vi "TDMS_NotesViewer.vi"() -> ()   [LabVIEW 2019]
panel:
  out "Experiment Notes":string
  in  "Files":i32(listbox)
  in  "Experiment Path":path
  in  "OK":bool
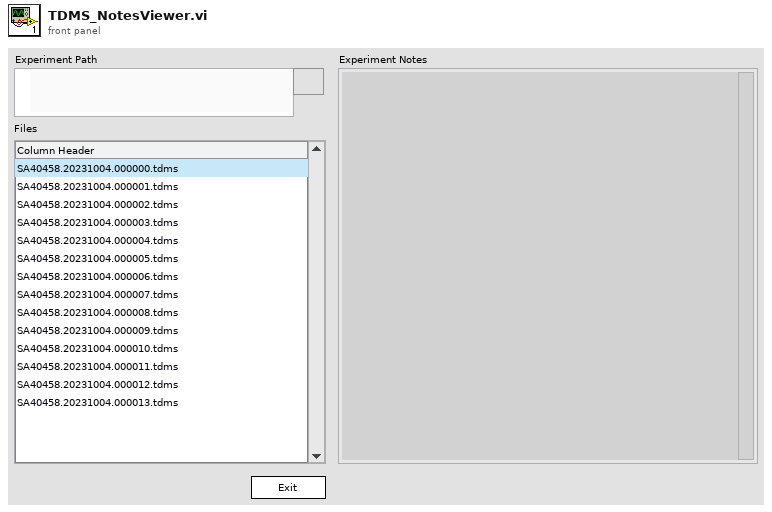
[diagram p1: front panel]
types:
  T1 = enum32{"Invalid", "Standard", "Closed", "Hidden", "Minimized", "Maximized"}
  T2 = enum32{"invalid app kind", "Development System", "Run Time System", "Student Edition", "Embedded LabVIEW", "Evaluation", "Custom"}
  T3 = cluster{"Core":cluster{"Current VI Reference":refnum<vi>, "Close Panel on Exit?":bool}, "Your Boolean data":bool, "Your string data":string, "File list":string[], "Experiment Path":path}
  T4 = cluster{"Current VI Reference":refnum<vi>, "Close Panel on Exit?":bool}
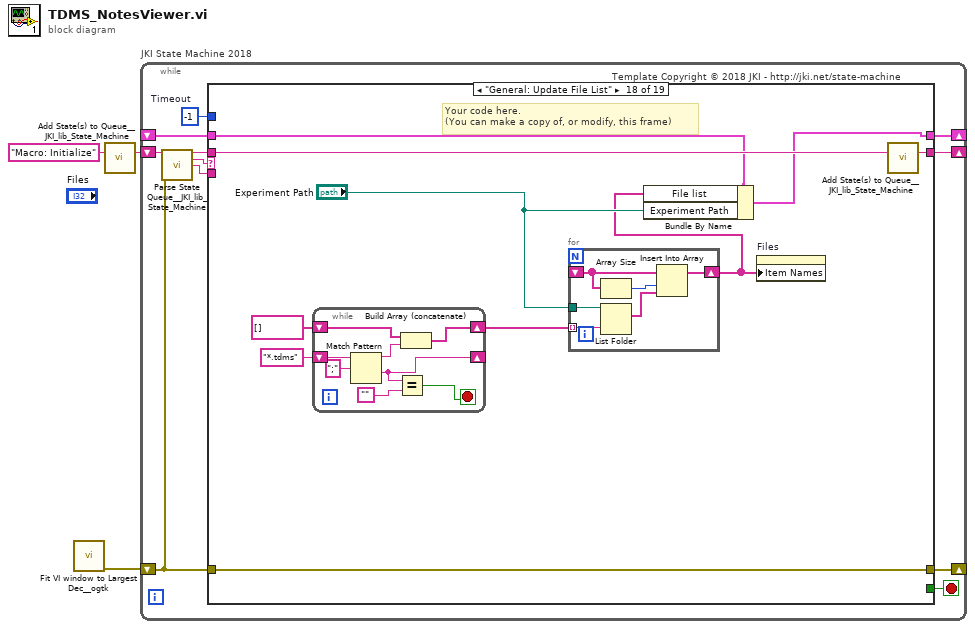
[diagram p0: block diagram]
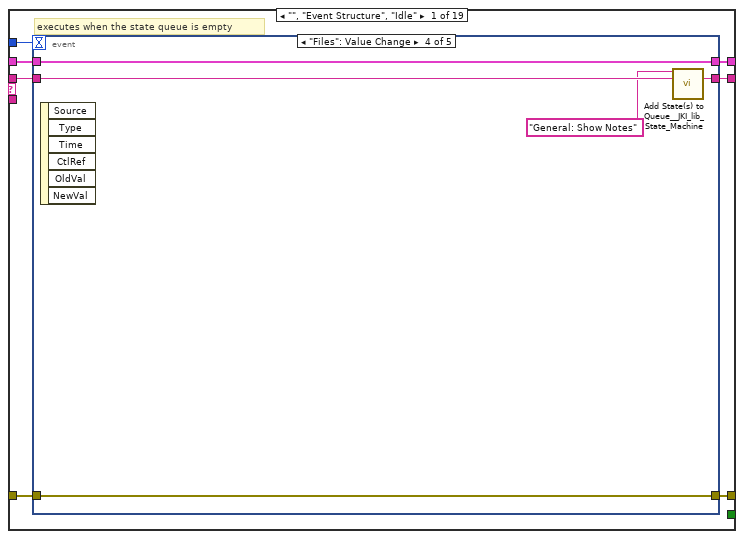
[diagram p2: hidden frame]
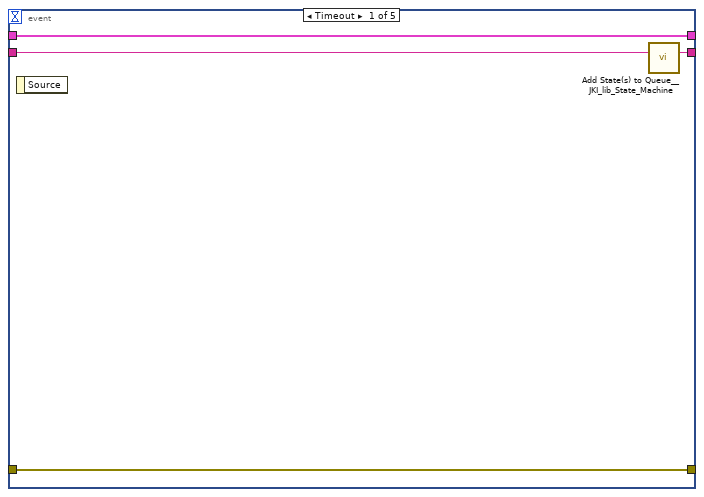
[diagram p3: hidden frame]
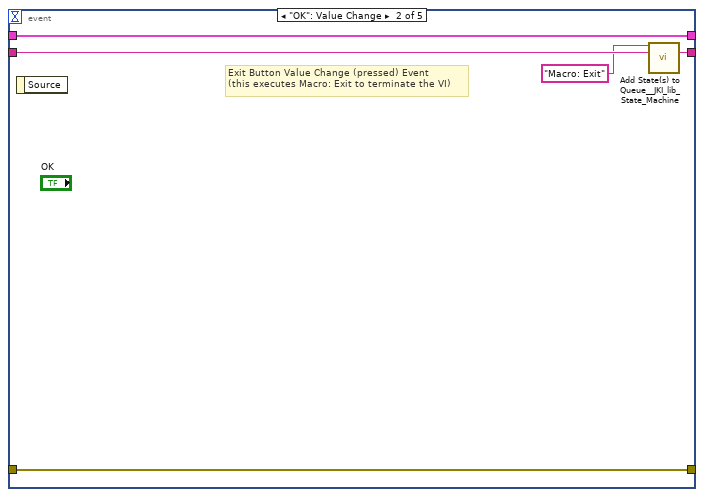
[diagram p4: hidden frame]
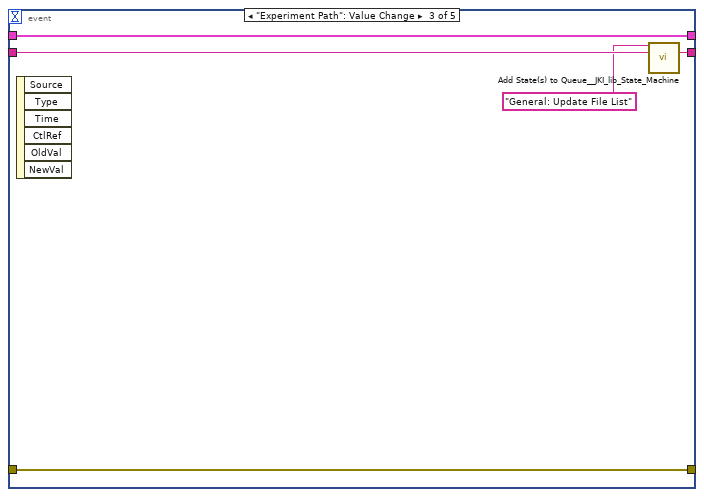
[diagram p5: hidden frame]
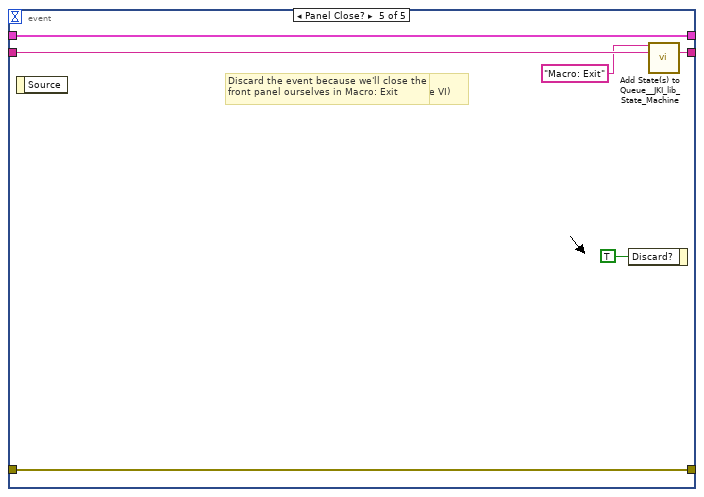
[diagram p6: hidden frame]
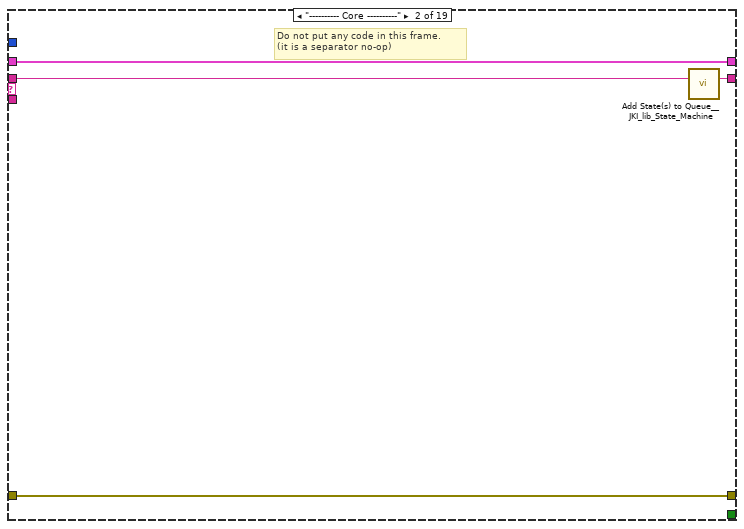
[diagram p7: hidden frame]
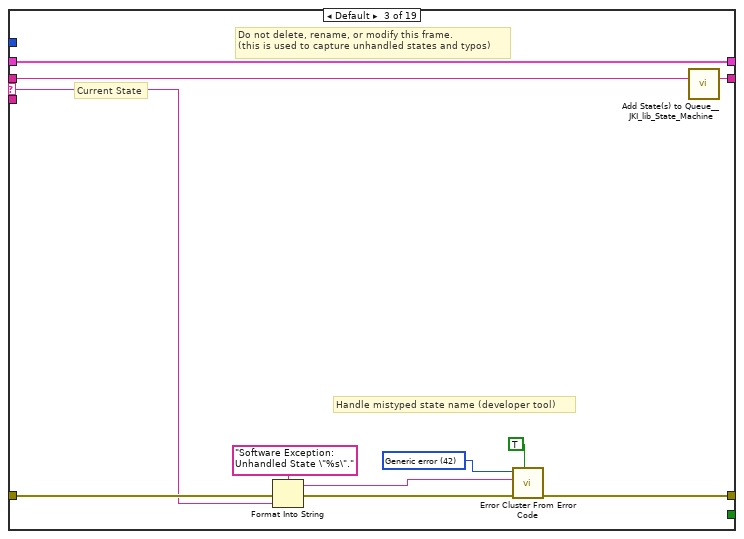
[diagram p8: hidden frame]
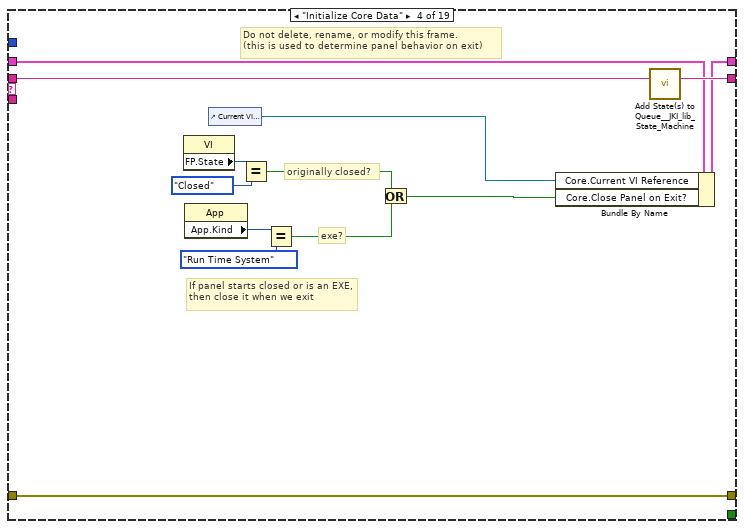
[diagram p9: hidden frame]
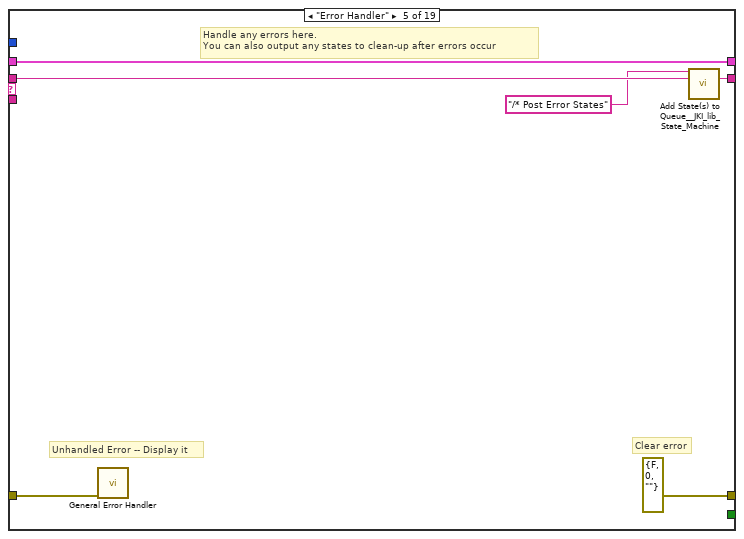
[diagram p10: hidden frame]
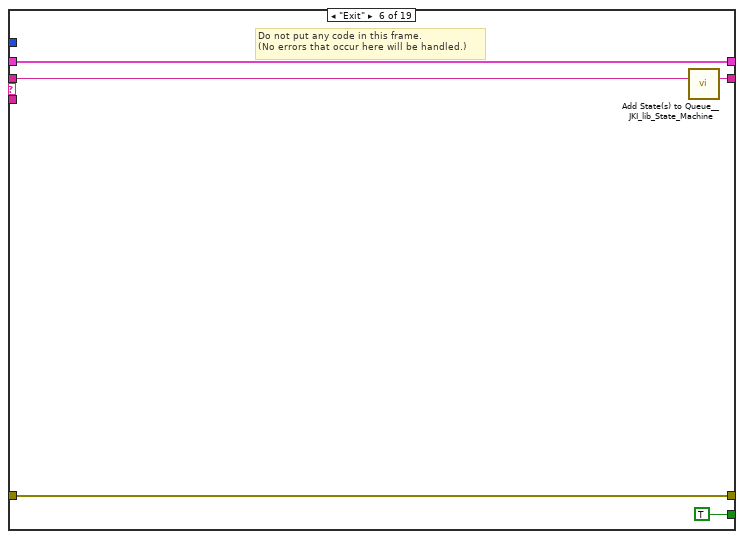
[diagram p11: hidden frame]
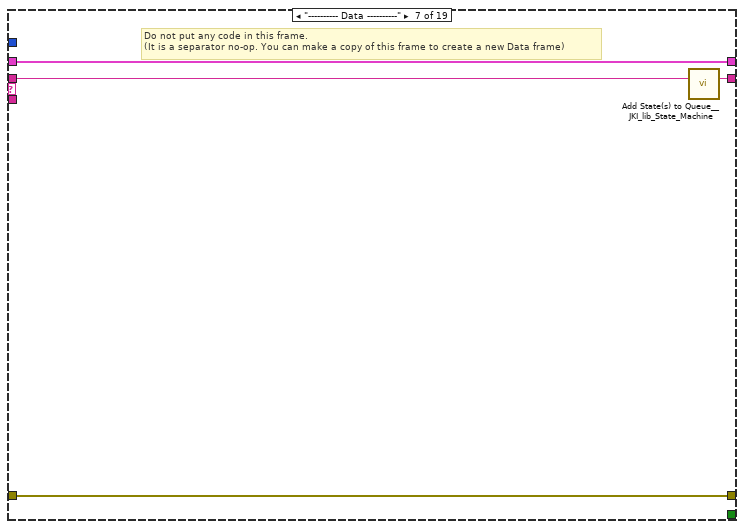
[diagram p12: hidden frame]
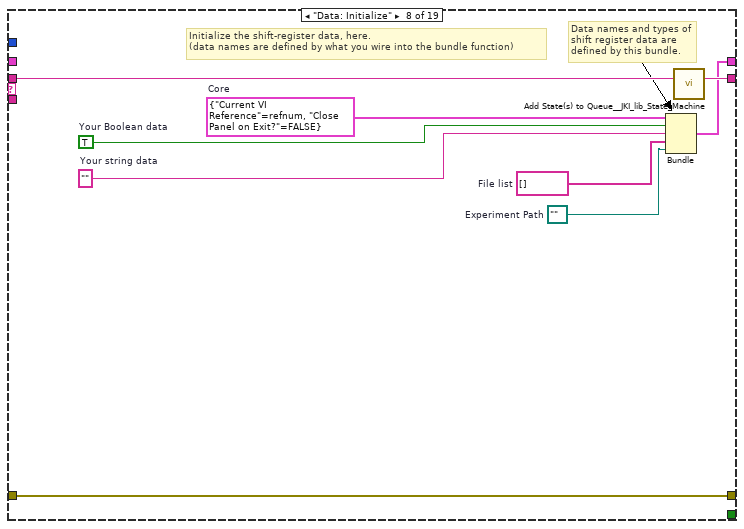
[diagram p13: hidden frame]
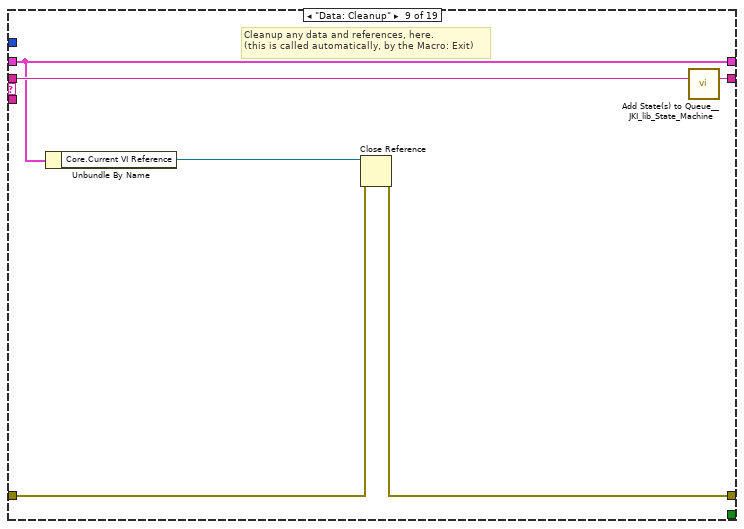
[diagram p14: hidden frame]
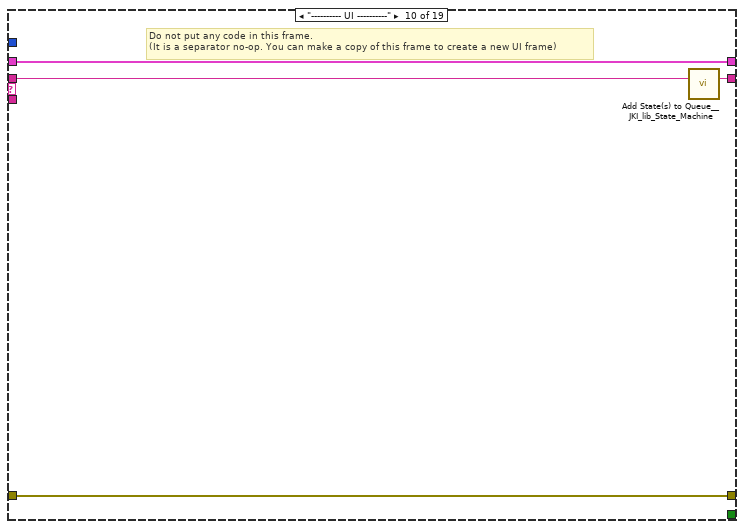
[diagram p15: hidden frame]
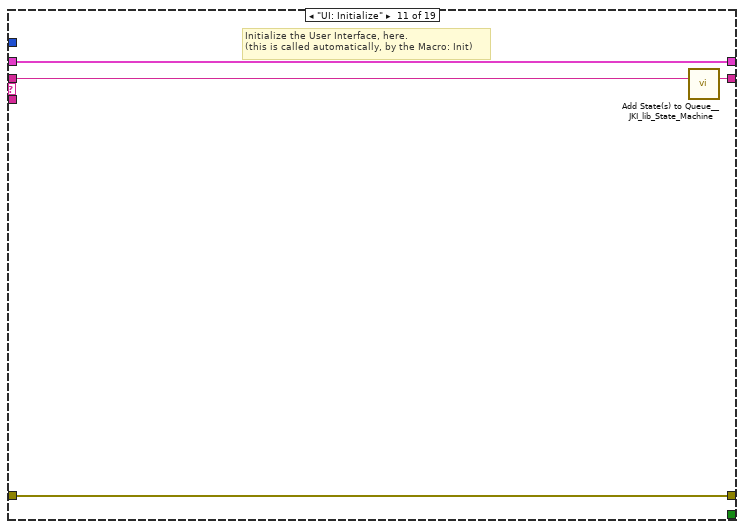
[diagram p16: hidden frame]
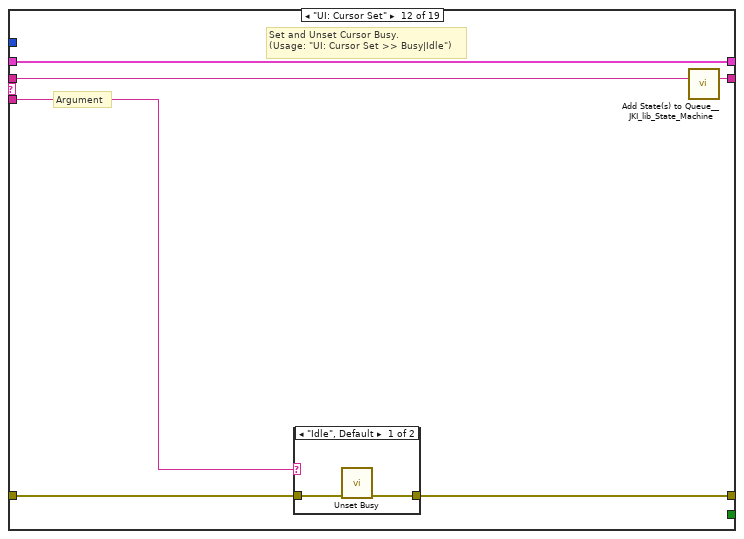
[diagram p17: hidden frame]
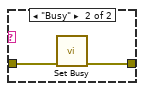
[diagram p18: hidden frame]
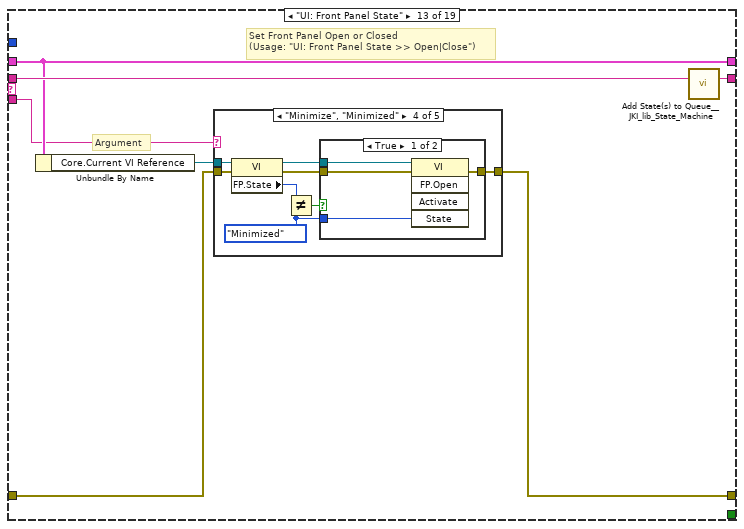
[diagram p19: hidden frame]
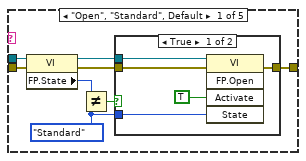
[diagram p20: hidden frame]
diagram:
  n1 = call <userlib>:"Fit VI window to Largest Dec__ogtk.vi"() -> ("error out"=w1:errorcluster)  [unwired: 6 in, 1 out]
  n2 = call <vilib>:"Add State(s) to Queue__JKI_lib_State_Machine.vi"("State(s) in (\"\")"="Macro: Initialize") -> ("States Out"=w3:string)  [unwired: 14 in]
  n3 = while "JKI State Machine 2018" {
    shift-right: [w7] -> _
    shift-left: _ -> [w6]
    shift-right: [w10] -> _
    shift-left: w1 -> [w4]
    shift-right: [w9] -> _
    shift-left: w3 -> [w11]
    stop <- w8 stop-if-true
    w5 = -1  # Timeout
    # "Template Copyright © 2018 JKI - http://jki.net/state-machine"
    n4 = call <vilib>:"Parse State Queue__JKI_lib_State_Machine.vi"("State Queue"=w11, "Error In (no error)"=w4) -> ("Remaining States"=w13:string, "Current State"=w14:string, "Arguments"=w12:string)  [unwired: 11 in]
    n5 = case shown="\"General: Update File List\"" w14 {
      selector: w14 -> [_ _ w51 _ _ _ _ _ _ _ _ _ _ _ _ _ _ _ _]
      tunnel: w13 -> [w21 w50 w55 w74 w80 w85 w89 w98 w104 w108 w112 w118 w129 w198 w203 w213 w217 w227 w259]
      tunnel: w12 -> [_ _ _ _ _ _ _ _ _ _ _ w113 w123 _ _ _ _ _ _]
      tunnel: w6 -> [w19 w47 w53 w67 w77 w83 w86 _ w99 w105 w110 w116 w125 w195 w200 w210 w214 w225 w256]
      tunnel: [w18 w48 w57 w71 errorcluster {"status"=FALSE, "code"=0, "source"=""} ("error out") w82 w87 w95 w100 w106 w109 w114 w126 w196 w201 w211 w215 w218 w257] -> w10
      tunnel: w4 -> [w17 w48 w56 w71 w76 w82 w87 w95 w101 w106 w109 w115 w127 w196 w201 w211 w215 w218 w257]
      tunnel: [w20 w49 w54 w73 w79 w84 w88 w97 w103 w107 w111 w117 w128 w197 w202 w212 w216 w226 w258] -> w9
      tunnel: [_ _ _ _ _ TRUE _ _ _ _ _ _ _ _ _ _ _ _ _] -> w8
      tunnel: [w16 w47 w53 w72 w77 w83 w86 w96 w99 w105 w110 w116 w125 w195 w200 w210 w214 w224 w256] -> w7
      tunnel: w5 -> [w15 _ _ _ _ _ _ _ _ _ _ _ _ _ _ _ _ _ _]
      frame "", "Event Structure", "Idle" {
        # "executes when the state queue is empty"
        n6 = event shown="[3] \"Files\": Value Change" {
          selector: _ -> [_ _ _ _ _]
          dyn-events: _ -> [_ _ _ _ _]
          timeout: w15 -> [_ _ _ _ _]
          tunnel: w21 -> [w25 w30 w35 w40 w46]
          tunnel: [w24 w29 w34 w39 w45] -> w20
          tunnel: w19 -> [w22 w27 w32 w37 w43]
          tunnel: [w23 w28 w33 w38 w44] -> w18
          tunnel: w17 -> [w23 w28 w33 w38 w44]
          tunnel: [w22 w27 w32 w37 w43] -> w16
          event Timeout {
            n7 = event-data() -> ()  [unwired: 1 in, 1 out]
            n8 = call <vilib>:"Add State(s) to Queue__JKI_lib_State_Machine.vi"("State(s) in (\"\")"=w25) -> ("States Out"=w24:string)  [unwired: 14 in]
          }
          event "OK": Value Change {
            # "Exit Button Value Change (pressed) Event\n(this executes Macro: Exit to terminate the VI)"
            n9 = event-data() -> ()  [unwired: 1 in, 1 out]
            n10 = call <vilib>:"Add State(s) to Queue__JKI_lib_State_Machine.vi"("State(s) in Front (\"\")"="Macro: Exit", "State(s) in (\"\")"=w30) -> ("States Out"=w29:string)  [unwired: 13 in]
          }
          event "Experiment Path": Value Change {
            n11 = event-data() -> ()  [unwired: 1 in, 6 out]
            n12 = call <vilib>:"Add State(s) to Queue__JKI_lib_State_Machine.vi"("State(s) in Front (\"\")"="General: Update File List", "State(s) in (\"\")"=w35) -> ("States Out"=w34:string)  [unwired: 13 in]
          }
          event "Files": Value Change {
            n13 = event-data() -> ()  [unwired: 1 in, 6 out]
            n14 = call <vilib>:"Add State(s) to Queue__JKI_lib_State_Machine.vi"("State(s) in Front (\"\")"="General: Show Notes", "State(s) in (\"\")"=w40) -> ("States Out"=w39:string)  [unwired: 13 in]
          }
          event Panel Close? {
            # "Discard the event because we'll close the front panel ourselves in Macro: Exit"
            # "Close Panel button (pressed) Event\n(this executes Macro: Exit to terminate the VI)"
            n15 = event-data() -> ()  [unwired: 1 in, 1 out]
            n16 = event-data("Discard?"=TRUE) -> ()  [unwired: 1 in, 1 out]
            n17 = call <vilib>:"Add State(s) to Queue__JKI_lib_State_Machine.vi"("State(s) in Front (\"\")"="Macro: Exit", "State(s) in (\"\")"=w46) -> ("States Out"=w45:string)  [unwired: 13 in]
          }
        }
      }
      frame "---------- Core ----------" {
        # "Do not put any code in this frame.\n(it is a separator no-op)"
        n18 = call <vilib>:"Add State(s) to Queue__JKI_lib_State_Machine.vi"("State(s) in (\"\")"=w50) -> ("States Out"=w49:string)  [unwired: 14 in]
      }
      frame Default {
        w60 = 42 items=["No error", "Argument error", "Memory is full", "Out of zone", "End of file", "File already open", "Generic file I/O error", "File not found", "File permission error", "Disk is full", "Duplicate path", "Too many files open", "System feature not enabled", "Resource file not found", "Cannot add resource", "Resource not found", "Image not found", "Image memory error", "Pen does not exist", "Config type invalid", "Config token not found", "Config parse error", "Config memory error", "Bad external code format", "Bad external code offset", "External code not present", "Null window", "Destroy window error", "Null menu", "Print aborted", "Bad print record", "Print driver error", "Windows error during printing", "Memory error during printing", "Print dialog error", "Generic print error", "Invalid device refnum", "Device not found", "Device parameter error", "Device unit error", "Cannot open device", "Device call aborted", "Generic error", "Cancelled by user", "Object ID too low", "Object ID too high", "Object not in heap", "Unknown heap", "Unknown object (invalid DefProc)", "Unknown object (DefProc not in table)", "Message out of range", "Invalid (null) method", "Unknown message", "Manager call not supported", "Bad address", "Network operation in progress", "Network operation timed out", "Connection is busy", "Network attribute not supported", "Network error", "Address in use", "System out of memory", "Connection aborted", "Connection refused", "Not connected", "Already connected", "Connection closed", "Initialization error (interapplication manager)", "Bad occurrence", "Wait on unbound occurrence handler", "Occurrence queue overflow", "Datalog type conflict", "Unused", "Unrecognized type (interapplication manager)", "Memory corrupt", "Failed to make temporary DLL", "Old CIN version", "Drag socket not found", "Failed to load drop-object", "Failed to register OLE object", "Failed to release OLE object", "Format specifier type mismatch", "Unknown format specifier", "Too few format specifiers", "Too many format specifiers", "Scan failed", "Newer CIN version", "Error converting to variant", "Runtime menu error", "Password tampered", "Variant attribute not found", "Incompatible variant data type", "Event data is not available", "Event Store is not present", "Occurrence is not found", "Event Queue is not created", "Event info is not available", "Refnum passed is NULL", "Error retrieving Class GUID", "Error retrieving CoClass GUID", "Error retrieving TypeLib GUID.", "Bad built application magic bytes.", "Specific driver is different from the specific driver associated with the Logical Name.", "There is no session opened to the class driver.", "Max Error", "MAX - Error with config objects", "MAX - Error loading configuration", "MAX - Group not supported"]
        # "Current State"
        # "Do not delete, rename, or modify this frame.\n(this is used to capture unhandled states and typos)"
        # "Handle mistyped state name (developer tool)"
        n19 = Format Into String(format string="Software Exception: Unhandled State \"%s\"." ("message"), error in=w56, w51) -> (resulting string=w59:string, error out=w58:errorcluster)  [unwired: 1 in]
        n20 = call <vilib>:"Error Cluster From Error Code.vi"("show call chain? (False)"=TRUE, "error in (no error)"=w58, "error message (\"\")"=w59, "error code (0)"=w60) -> ("error out"=w57:errorcluster)  [unwired: 5 in]
        n21 = call <vilib>:"Add State(s) to Queue__JKI_lib_State_Machine.vi"("State(s) in (\"\")"=w55) -> ("States Out"=w54:string)  [unwired: 14 in]
      }
      frame "Initialize Core Data" {
        # "Do not delete, rename, or modify this frame.\n(this is used to determine panel behavior on exit)"
        # "originally closed?"
        # "exe?"
        # "If panel starts closed or is an EXE, then close it when we exit"
        n22 = property class="VI"() -> ("FP.State"=w64:T1)  [unwired: 2 in, 2 out]
        n23 = property class="App"() -> ("App.Kind"=w70:T2)  [unwired: 2 in, 2 out]
        n24 = control-ref of="Current VI Reference"() -> (w65:refnum<vi>)
        n25 = Equal?(x=w64, y=T1."Closed" ("Front Panel Window:State")) -> (x = y?=w62:bool)
        n26 = Equal?(x=w70, y=T2."Run Time System" ("Application:Kind")) -> (x = y?=w68:bool)
        n27 = Or(x=w62, y=w68) -> (x .or. y?=w66:bool)
        n28 = Bundle By Name(cluster=w67, "Core.Current VI Reference"=w65, "Core.Close Panel on Exit?"=w66) -> (w72:T3)
        n29 = call <vilib>:"Add State(s) to Queue__JKI_lib_State_Machine.vi"("State(s) in (\"\")"=w74) -> ("States Out"=w73:string)  [unwired: 14 in]
      }
      frame "Error Handler" {
        # "Unhandled Error -- Display it"
        # "Handle any errors here.\nYou can also output any states to clean-up after errors occur"
        # "Clear error"
        n30 = call <vilib>:"General Error Handler.vi"("error in (no error)"=w76) -> ()  [unwired: 10 in, 5 out]
        n31 = call <vilib>:"Add State(s) to Queue__JKI_lib_State_Machine.vi"("State(s) in Front (\"\")"="/* Post Error States", "State(s) in (\"\")"=w80) -> ("States Out"=w79:string)  [unwired: 13 in]
      }
      frame "Exit" {
        # "Do not put any code in this frame.\n(No errors that occur here will be handled.)"
        n32 = call <vilib>:"Add State(s) to Queue__JKI_lib_State_Machine.vi"("State(s) in (\"\")"=w85) -> ("States Out"=w84:string)  [unwired: 14 in]
      }
      frame "---------- Data ----------" {
        # "Do not put any code in this frame.\n(It is a separator no-op. You can make a copy of this frame to create a new Data frame)"
        n33 = call <vilib>:"Add State(s) to Queue__JKI_lib_State_Machine.vi"("State(s) in (\"\")"=w89) -> ("States Out"=w88:string)  [unwired: 14 in]
      }
      frame "Data: Initialize" {
        w90 = path ""  # Experiment Path
        w91 = string[] []  # File list
        w92 = T4 {"Current VI Reference"=refnum, "Close Panel on Exit?"=FALSE}  # Core
        w94 = TRUE  # Your Boolean data
        w93 = ""  # Your string data
        # "Data names and types of shift register data are defined by this bundle."
        # "Initialize the shift-register data, here.\n(data names are defined by what you wire into the bundle function)"
        n34 = Bundle("Core"=w92, "Your Boolean data"=w94, "Your string data"=w93, "File list"=w91, "Experiment Path"=w90) -> (w96:T3)  [unwired: 1 in]
        n35 = call <vilib>:"Add State(s) to Queue__JKI_lib_State_Machine.vi"("State(s) in (\"\")"=w98) -> ("States Out"=w97:string)  [unwired: 14 in]
      }
      frame "Data: Cleanup" {
        # "Cleanup any data and references, here.\n(this is called automatically, by the Macro: Exit)"
        n36 = Unbundle By Name(w99) -> ("Core.Current VI Reference"=w102:refnum<vi>)
        n37 = Close Reference(reference=w102, error in (no error)=w101) -> (error out=w100:errorcluster)
        n38 = call <vilib>:"Add State(s) to Queue__JKI_lib_State_Machine.vi"("State(s) in (\"\")"=w104) -> ("States Out"=w103:string)  [unwired: 14 in]
      }
      frame "---------- UI ----------" {
        # "Do not put any code in this frame.\n(It is a separator no-op. You can make a copy of this frame to create a new UI frame)"
        n39 = call <vilib>:"Add State(s) to Queue__JKI_lib_State_Machine.vi"("State(s) in (\"\")"=w108) -> ("States Out"=w107:string)  [unwired: 14 in]
      }
      frame "UI: Initialize" {
        # "Initialize the User Interface, here.\n(this is called automatically, by the Macro: Init)"
        n40 = call <vilib>:"Add State(s) to Queue__JKI_lib_State_Machine.vi"("State(s) in (\"\")"=w112) -> ("States Out"=w111:string)  [unwired: 14 in]
      }
      frame "UI: Cursor Set" {
        # "Argument"
        # "Set and Unset Cursor Busy.\n(Usage: \"UI: Cursor Set >> Busy|Idle\")"
        n41 = case shown="\"Idle\", Default" w113 {
          tunnel: w115 -> [w120 w122]
          tunnel: [w119 w121] -> w114
          frame "Idle", Default {
            n42 = call <vilib>:"Unset Busy.vi"("error in (no error)"=w120) -> ("error out"=w119:errorcluster)  [unwired: 10 in]
          }
          frame "Busy" {
            n43 = call <vilib>:"Set Busy.vi"("error in (no error)"=w122) -> ("error out"=w121:errorcluster)  [unwired: 9 in, 1 out]
          }
        }
        n44 = call <vilib>:"Add State(s) to Queue__JKI_lib_State_Machine.vi"("State(s) in (\"\")"=w118) -> ("States Out"=w117:string)  [unwired: 14 in]
      }
      frame "UI: Front Panel State" {
        # "Argument"
        # "Set Front Panel Open or Closed\n(Usage: \"UI: Front Panel State >> Open|Close\")"
        n45 = Unbundle By Name(w125) -> ("Core.Current VI Reference"=w124:refnum<vi>)
        n46 = case shown="\"Minimize\", \"Minimized\"" w123 {
          tunnel: w127 -> [w135 w150 w161 w174 w187]
          tunnel: [w137 w151 w163 w176 w189] -> w126
          tunnel: w124 -> [w136 w148 w162 w175 w188]
          frame "Open", "Standard", Default {
            w130 = T1."Standard" ("State")
            n47 = property class="VI"(reference=w136, error in=w135) -> (reference out=w133:refnum<vi>, error out=w134:errorcluster, "FP.State"=w132:T1)
            n48 = Not Equal?(x=w132, y=w130) -> (x != y?=w131:bool)
            n49 = case shown="True" w131 {
              tunnel: [w141 w143] -> w137
              tunnel: w134 -> [w140 w143]
              tunnel: w133 -> [w139 _]
              tunnel: w130 -> [w138 _]
              frame True {
                n50 = invoke class="VI" method="FP.Open"(reference=w139, error in=w140, "Activate"=TRUE, "State"=w138) -> (error out=w141:errorcluster)  [unwired: 1 in, 4 out]
              }
              frame False {
              }
            }
          }
          frame "Close", "Closed" {
            n51 = property class="VI"(reference=w148, error in=w150) -> (reference out=w147:refnum<vi>, error out=w149:errorcluster, "FP.State"=w145:T1)
            n52 = Not Equal?(x=w145, y=T1."Closed" ("Front Panel Window:State")) -> (x != y?=w144:bool)
            n53 = case shown="True" w144 {
              tunnel: [w152 w155] -> w151
              tunnel: w149 -> [w152 w154]
              tunnel: w147 -> [_ w153]
              frame False {
              }
              frame True {
                n54 = invoke class="VI" method="FP.Close"(reference=w153, error in=w154) -> (error out=w155:errorcluster)  [unwired: 1 in, 2 out]
              }
            }
          }
          frame "Hidden", "Hide" {
            w156 = T1."Hidden" ("State")
            n55 = property class="VI"(reference=w162, error in=w161) -> (reference out=w159:refnum<vi>, error out=w160:errorcluster, "FP.State"=w158:T1)
            n56 = Not Equal?(x=w158, y=w156) -> (x != y?=w157:bool)
            n57 = case shown="True" w157 {
              tunnel: [w167 w168] -> w163
              tunnel: w160 -> [w166 w168]
              tunnel: w159 -> [w165 _]
              tunnel: w156 -> [w164 _]
              frame True {
                n58 = invoke class="VI" method="FP.Open"(reference=w165, error in=w166, "State"=w164) -> (error out=w167:errorcluster)  [unwired: 2 in, 4 out]
              }
              frame False {
              }
            }
          }
          frame "Minimize", "Minimized" {
            w169 = T1."Minimized" ("State")
            n59 = property class="VI"(reference=w175, error in=w174) -> (reference out=w172:refnum<vi>, error out=w173:errorcluster, "FP.State"=w171:T1)
            n60 = Not Equal?(x=w171, y=w169) -> (x != y?=w170:bool)
            n61 = case shown="True" w170 {
              tunnel: [w180 w181] -> w176
              tunnel: w173 -> [w179 w181]
              tunnel: w172 -> [w178 _]
              tunnel: w169 -> [w177 _]
              frame True {
                n62 = invoke class="VI" method="FP.Open"(reference=w178, error in=w179, "State"=w177) -> (error out=w180:errorcluster)  [unwired: 2 in, 4 out]
              }
              frame False {
              }
            }
          }
          frame "Maximize", "Maximized" {
            w182 = T1."Maximized" ("State")
            n63 = property class="VI"(reference=w188, error in=w187) -> (reference out=w185:refnum<vi>, error out=w186:errorcluster, "FP.State"=w184:T1)
            n64 = Not Equal?(x=w184, y=w182) -> (x != y?=w183:bool)
            n65 = case shown="True" w183 {
              tunnel: [w193 w194] -> w189
              tunnel: w186 -> [w192 w194]
              tunnel: w185 -> [w191 _]
              tunnel: w182 -> [w190 _]
              frame True {
                n66 = invoke class="VI" method="FP.Open"(reference=w191, error in=w192, "State"=w190) -> (error out=w193:errorcluster)  [unwired: 2 in, 4 out]
              }
              frame False {
              }
            }
          }
        }
        n67 = call <vilib>:"Add State(s) to Queue__JKI_lib_State_Machine.vi"("State(s) in (\"\")"=w129) -> ("States Out"=w128:string)  [unwired: 14 in]
      }
      frame "---------- Macro ----------" {
        # "Do not put any code in this frame.\n(It is a separator no-op. You can make a copy of this frame to create a new Macro frame)"
        n68 = call <vilib>:"Add State(s) to Queue__JKI_lib_State_Machine.vi"("State(s) in (\"\")"=w198) -> ("States Out"=w197:string)  [unwired: 14 in]
      }
      frame "Macro: Initialize" {
        w199 = "Data: Initialize\nInitialize Core Data\nUI: Initialize\nUI: Front Panel State >> Open\nGeneral: Update File List"  # Data: Initialize Initialize Core Data UI: Initialize UI: Front Panel State >> Open General: Update File List
        # "Initialization Macro\n(This is called once, when the VI starts)"
        n69 = call <vilib>:"Add State(s) to Queue__JKI_lib_State_Machine.vi"("State(s) in Front (\"\")"=w199, "State(s) in (\"\")"=w203) -> ("States Out"=w202:string)  [unwired: 13 in]
      }
      frame "Macro: Exit" {
        # "Exit Macro\n(This is called once, when the VI exits)"
        n70 = Unbundle By Name(w210) -> ("Core.Close Panel on Exit?"=w209:bool)
        n71 = Select(t="UI: Front Panel State >> Close", s=w209, f="") -> (s? t:f=w206:string)
        n72 = call <vilib>:"Add State(s) to Queue__JKI_lib_State_Machine.vi"("State(s) in (\"\")"=w206, "State(s) at Back (\"\")"="Data: Cleanup\nExit") -> ("States Out"=w204:string)  [unwired: 13 in]
        n73 = call <vilib>:"Add State(s) to Queue__JKI_lib_State_Machine.vi"("State(s) in Front (\"\")"=w204, "State(s) in (\"\")"=w213) -> ("States Out"=w212:string)  [unwired: 13 in]
      }
      frame "---------- General ----------" {
        # "Template Separator\n(You can make a copy of, or modify, this frame)"
        n74 = call <vilib>:"Add State(s) to Queue__JKI_lib_State_Machine.vi"("State(s) in (\"\")"=w217) -> ("States Out"=w216:string)  [unwired: 14 in]
      }
      frame "General: Update File List" {
        # "Your code here.\n(You can make a copy of, or modify, this frame)"
        n75 = while {
          shift-right: [w228] -> _
          shift-left: "*.tdms" ("pattern") -> [w234]
          shift-right: [w229] -> w222
          shift-left: string[] [] -> [w231]
          stop <- w232 stop-if-true
          n76 = Match Pattern(string=w234, regular expression=";" ("search string/char (-)")) -> (before substring=w230:string, after substring=w228:string)  [unwired: 1 in, 2 out]
          n77 = Equal?(x=w228, y="") -> (x = y?=w232:bool)
          n78 = Build Array (concatenate)(w231, w230) -> (w229:string[])
        }
        n79 = for {
          tunnel: w222 -> [w241] mode=indexing
          shift-right: [w240] -> w219
          shift-left: _ -> [w238]
          tunnel: "Experiment Path" -> [w236]
          n80 = Array Size(array=w238) -> (size(s)=w237:i32)
          n81 = List Folder(path=w236, pattern=w241) -> (filenames=w239:string[])  [unwired: 2 in, 3 out]
          n82 = Insert Into Array(array=w238, index=w237, new element=w239) -> (w240:string[])
        }
        n83 = Bundle By Name(cluster=w225, "File list"=w219, "Experiment Path"="Experiment Path") -> (w224:T3)
        n84 = property on="Files" class="LstBox (strict)"("Item Names"=w219) -> ()  [unwired: 2 in, 2 out]
        n85 = call <vilib>:"Add State(s) to Queue__JKI_lib_State_Machine.vi"("State(s) in (\"\")"=w227) -> ("States Out"=w226:string)  [unwired: 14 in]
      }
      frame "General: Show Notes" {
        # "Your code here.\n(You can make a copy of, or modify, this frame)"
        n86 = Unbundle By Name(w256) -> ("Experiment Path"=w254:path, "File list"=w255:string[])
        n87 = local read "Files"() -> (w252:i32)
        n88 = Path To String(path=w254) -> (string=w253:string)
        n89 = Index Array(array=w255, index=w252) -> (element=w250:string)
        n90 = Concatenate Strings(w253, "\\" ("string"), w250) -> (w251:string)
        n91 = String To Path(string=w251) -> (path=w248:path)
        n92 = TDMS Open(11:w248) -> (0:w247:errorcluster, 3:w246:refnum<k34>)  [unwired: 6 in]
        n93 = TDMS Get Properties(5:"" ("data type"), 7:"Notes" ("property name"), 8:w247, 11:w246) -> (4:→"Experiment Notes":string)  [unwired: 2 in, 5 out]
        n94 = property on="Experiment Notes" class="Str"("VScrollVis"=TRUE ("Vertical Scrollbar Visible")) -> ()  [unwired: 2 in, 2 out]
        n95 = call <vilib>:"Add State(s) to Queue__JKI_lib_State_Machine.vi"("State(s) in (\"\")"=w259) -> ("States Out"=w258:string)  [unwired: 14 in]
      }
    }
  }
